vi "CRYLoad Hardware Calibration.vi"() -> ()   [LabVIEW 2013]
uses:
  CRYSystem/Typedef Control/CRYStep.ctl
  CRYSystem/Typedef Control/CRYCalibration 2DCluster.ctl
  CRYSystem/Typedef Control/CRYCalibration Cluster.ctl
  CRYSystem/Typedef Control/CRYData Cluster.ctl
  CRYProject Editor Global.vi
  CRYMainGlobal.vi
panel:
  in  "Step":T1 {"Repeat State Array"."Start" format="%#_5g"; "Y dB ref" format="%.1f"; "Y data" items=["dB", "Lin"]; "Start" format="%#_5g"}
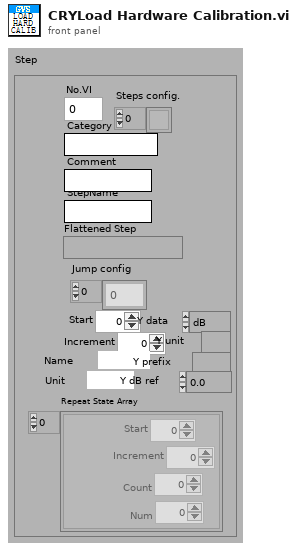
[diagram p1: front panel]
types:
  T1 = typedef "CRYStep.ctl" = cluster{"No.VI":i32, "Category":string, "StepName":string, "Seq setup flattened":string, "Comment":string, "Steps config.":bool[], "Jump config":i32[], "Start":dbl, "Increment":dbl, "Name":string, "Unit":string, "Y data":u16, "Y prefix":string, "Y dB ref":dbl, "Y unit":string, "Repeat State Array":cluster{"Start":dbl, "Increment":dbl, "Count":i32, "Num":i32}[]}
  T2 = typedef "CRYCalibration All Cluster.ctl" = cluster{"Calibration 2D":T3[], "Help":string, "Tab Value":i32, "Input Signal Type":string, "Output Signal Type":string}
  T3 = typedef "CRYCalibration 2DCluster.ctl" = cluster{"Calibration":T4, "Corr Curve":T5, "EQ Curve":T5, "Sens Curve":T5}
  T4 = typedef "CRYCalibration Cluster.ctl" = cluster{"Calibration Step Name":string, "Device":string, "Correction Curve Name":string, "Equalization Curve Name":string, "Sensitivity Curve Name":string, "Corr Folder and File":string, "EQ Folder and File":string, "Sens Folder and File":string, "Corr Step size":u16, "EQ Step size":u16, "Input":bool, "Last Cal Date (sec)":timestamp, "Cha Name":string, "Corr Curve Found":bool, "EQ Curve Found":bool, "Sens Curve Found":bool, "Signal Type":string, "Calibrated Device":string, "Hz":u32}
  T5 = typedef "CRYData Cluster.ctl" = cluster{"Name":string, "Curve":cluster{"x":dbl, "y":dbl, "z":dbl}[], "X data":u16, "Y data":u16, "Z data":u16, "X axis":u16, "Y axis":u16, "Z axis":u16, "X unit":string, "Y unit":string, "Z unit":string, "X dB ref":dbl, "Y dB ref":dbl, "Z dB ref":dbl, "single val":bool, "protected":bool, "display X":bool, "display Y":bool, "display Z":bool, "Test Info":string, "Step No.":i32, "Plot Settings":cluster{"Color":u32, "Interpolation":u8, "Point Style":u8, "Line Style":u8, "Point Color":u32, "Line Width":u8, "Bar Plot Style":u8, "Fill To":i16}, "AutoProtect":bool}
  T6 = cluster{"Signal Type":string, "Calibrated Device":string, "Cha Name":string, "Input":bool}[]
  T7 = typedef "CRYHardware.ctl" = cluster{"Name":string, "Analog I/O":u16, "Digital I/O":u16, "Channels":u8, "Dig Dev ID":u8, "N ports":u8, "Interface":u32, "Dig I/O Ports":cluster{"port #":i16, "width":i16, "direction":i32}[], "Interf settings":cluster{"Type":u16, "COM Port":u8, "Baud rate":u32, "Data bits":u32, "Parity":u16, "Stop bits":u16, "Flow control":u16, "Dev ID IEEE":u8}[], "N interfs":i32, "udev SNs":i16[], "udev enable":bool, "Channel Array":T8[], "Cal sequence":string, "SelectedIn":u16, "SelectedOut":u16, "SelectedTab":u16, "State":bool, "Help":string, "Advanced":bool, "In Audio Driver":u16, "Out Audio Driver":u16}
  T8 = typedef "CRYHardware Channel Info.ctl" = cluster{"ID":i32, "Name":string, "Digital":bool, "Input":bool, "Device Name":string, "Hardware Ch ID":u8, "Vmax (V)":dbl, "Latency (samples)":dbl, "Sampling Rate (Hz)":u32, "Bit Depth":u32, "Anti-aliasing Factor (%fs)":sgl, "DAQmx Channel":tag, "term config":i32, "Coupling":i32, "IEPE en":bool, "ASIOChannel Name":string, "Audio Driver":u16, "ASIOChannel Index":u8}
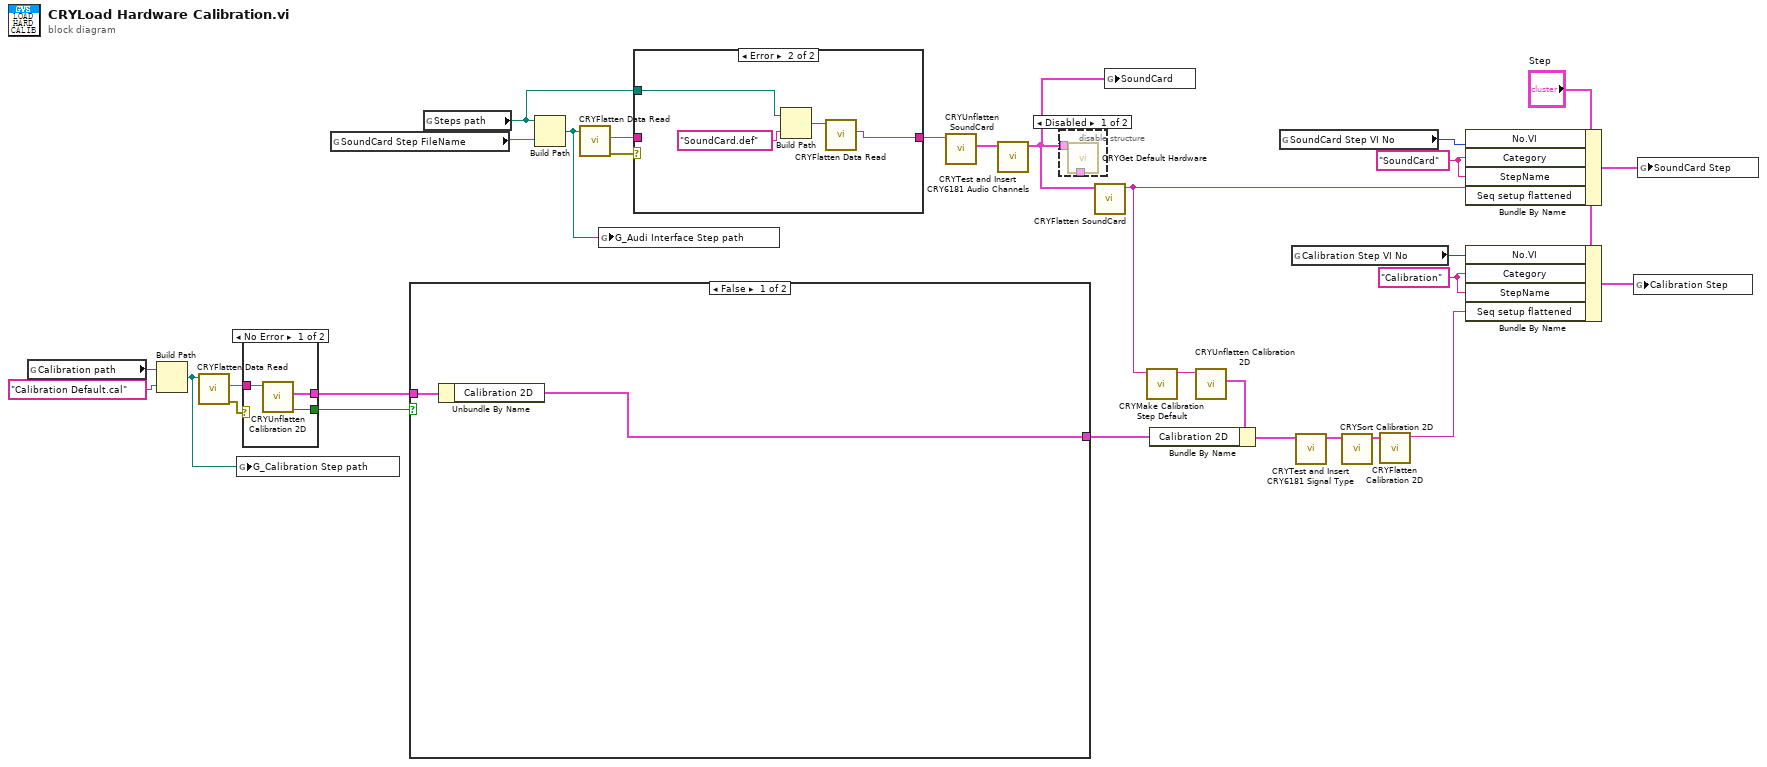
[diagram p0: block diagram]
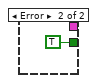
[diagram p4: hidden frame]
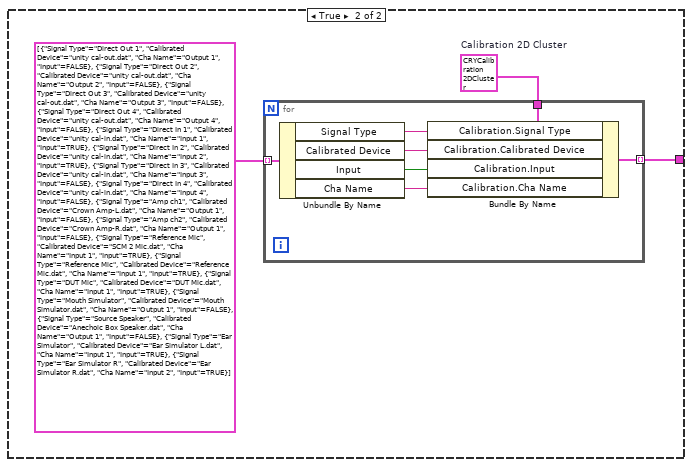
[diagram p5: hidden frame]
diagram:
  w30 = "Calibration" ("CategoryName")
  w29 = "SoundCard" ("CategoryName")
  n1 = global read "CRYMainGlobal.vi" "Calibration path"() -> (w14:path)
  n2 = Build Path(base path=w14, name or relative path="Calibration Default.cal") -> (appended path=w8:path)
  n3 = call "CRYFlatten Data Read.vi"("Path In"=w8) -> ("error out"=w15:errorcluster, "Flatten Data Out"=w19:string)  [unwired: 6 in, 1 out]
  n4 = global write "CRYProject Editor Global.vi" "G_Calibration Step path"(w8) -> ()
  n5 = case shown="No Error" w15 {
    tunnel: w19 -> [w33 _]
    tunnel: [w32 TRUE ("Error?")] -> w18
    tunnel: [w31 _] -> w17
    frame No Error {
      n6 = call "CRYUnflatten Calibration 2D.vi"("Flattened Calibration"=w33) -> ("Error?"=w32:bool, "Calibration Step Out"=w31:T2)  [unwired: 2 in, 7 out]
    }
    frame Error {
    }
  }
  n7 = global read "CRYMainGlobal.vi" "SoundCard Step FileName"() -> (w1:string)
  n8 = case shown="False" w18 {
    tunnel: w17 -> [w36 _]
    tunnel: [w35 w37] -> w16
    frame False {
      n9 = Unbundle By Name(w36) -> ("Calibration 2D"=w35:T3[])
    }
    frame True {
      w39 = T3 {"Calibration"={"Calibration Step Name"="", "Device"="", "Correction Curve Name"="", "Equalization Curve Name"="", "Sensitivity Curve Name"="", "Corr Folder and File"="", "EQ Folder and File"="", "Sens Folder and File"="", "Corr Step size"=0, "EQ Step size"=0, "Input"=FALSE, "Last Cal Date (sec)"=timestamp(0 s since 1904-01-01), "Cha Name"="", "Corr Curve Found"=FALSE, "EQ Curve Found"=FALSE, "Sens Curve Found"=FALSE, "Signal Type"="", "Calibrated Device"="", "Hz"=0}, "Corr Curve"={"Name"="", "Curve"=[], "X data"=1, "Y data"=1, "Z data"=1, "X axis"=0, "Y axis"=1, "Z axis"=1, "X unit"="Hz", "Y unit"="", "Z unit"="deg.", "X dB ref"=1.0, "Y dB ref"=1.0, "Z dB ref"=1.0, "single val"=FALSE, "protected"=FALSE, "display X"=TRUE, "display Y"=TRUE, "display Z"=TRUE, "Test Info"="", "Step No."=0, "Plot Settings"={"Color"=0, "Interpolation"=0, "Point Style"=0, "Line Style"=0, "Point Color"=0, "Line Width"=0, "Bar Plot Style"=0, "Fill To"=0}, "AutoProtect"=FALSE}, "EQ Curve"={"Name"="", "Curve"=[], "X data"=1, "Y data"=1, "Z data"=1, "X axis"=0, "Y axis"=1, "Z axis"=1, "X unit"="Hz", "Y unit"="", "Z unit"="deg.", "X dB ref"=1.0, "Y dB ref"=1.0, "Z dB ref"=1.0, "single val"=FALSE, "protected"=FALSE, "display X"=TRUE, "display Y"=TRUE, "display Z"=TRUE, "Test Info"="", "Step No."=0, "Plot Settings"={"Color"=0, "Interpolation"=0, "Point Style"=0, "Line Style"=0, "Point Color"=0, "Line Width"=0, "Bar Plot Style"=0, "Fill To"=0}, "AutoProtect"=FALSE}, "Sens Curve"={"Name"="", "Curve"=[], "X data"=1, "Y data"=1, "Z data"=1, "X axis"=0, "Y axis"=1, "Z axis"=1, "X unit"="Hz", "Y unit"="", "Z unit"="deg.", "X dB ref"=1.0, "Y dB ref"=1.0, "Z dB ref"=1.0, "single val"=FALSE, "protected"=FALSE, "display X"=TRUE, "display Y"=TRUE, "display Z"=TRUE, "Test Info"="", "Step No."=0, "Plot Settings"={"Color"=0, "Interpolation"=0, "Point Style"=0, "Line Style"=0, "Point Color"=0, "Line Width"=0, "Bar Plot Style"=0, "Fill To"=0}, "AutoProtect"=FALSE}}  # Calibration 2D Cluster
      n10 = for {
        tunnel: T6 [{"Signal Type"="Direct Out 1", "Calibrated Device"="unity cal-out.dat", "Cha Name"="Output 1", "Input"=FALSE}, {"Signal Type"="Direct Out 2", "Calibrated Device"="unity cal-out.dat", "Cha Name"="Output 2", "Input"=FALSE}, {"Signal Type"="Direct Out 3", "Calibrated Device"="unity cal-out.dat", "Cha Name"="Output 3", "Input"=FALSE}, {"Signal Type"="Direct Out 4", "Calibrated Device"="unity cal-out.dat", "Cha Name"="Output 4", "Input"=FALSE}, {"Signal Type"="Direct In 1", "Calibrated Device"="unity cal-in.dat", "Cha Name"="Input 1", "Input"=TRUE}, {"Signal Type"="Direct In 2", "Calibrated Device"="unity cal-in.dat", "Cha Name"="Input 2", "Input"=TRUE}, {"Signal Type"="Direct In 3", "Calibrated Device"="unity cal-in.dat", "Cha Name"="Input 3", "Input"=FALSE}, {"Signal Type"="Direct In 4", "Calibrated Device"="unity cal-in.dat", "Cha Name"="Input 4", "Input"=FALSE}, {"Signal Type"="Amp ch1", "Calibrated Device"="Crown Amp-L.dat", "Cha Name"="Output 1", "Input"=FALSE}, {"Signal Type"="Amp ch2", "Calibrated Device"="Crown Amp-R.dat", "Cha Name"="Output 1", "Input"=FALSE}, {"Signal Type"="Reference Mic", "Calibrated Device"="SCM 2 Mic.dat", "Cha Name"="Input 1", "Input"=TRUE}, {"Signal Type"="Reference Mic", "Calibrated Device"="Reference Mic.dat", "Cha Name"="Input 1", "Input"=TRUE}, {"Signal Type"="DUT Mic", "Calibrated Device"="DUT Mic.dat", "Cha Name"="Input 1", "Input"=TRUE}, {"Signal Type"="Mouth Simulator", "Calibrated Device"="Mouth Simulator.dat", "Cha Name"="Output 1", "Input"=FALSE}, {"Signal Type"="Source Speaker", "Calibrated Device"="Anechoic Box Speaker.dat", "Cha Name"="Output 1", "Input"=FALSE}, {"Signal Type"="Ear Simulator", "Calibrated Device"="Ear Simulator L.dat", "Cha Name"="Input 1", "Input"=TRUE}, {"Signal Type"="Ear Simulator R", "Calibrated Device"="Ear Simulator R.dat", "Cha Name"="Input 2", "Input"=TRUE}] ("Array") -> [w46] mode=indexing
        tunnel: w39 -> [w45]
        tunnel: [w40] -> w37 mode=indexing
        n11 = Unbundle By Name(w46) -> ("Signal Type"=w41:string, "Calibrated Device"=w42:string, "Input"=w43:bool, "Cha Name"=w44:string)
        n12 = Bundle By Name(cluster=w45, "Calibration.Signal Type"=w41, "Calibration.Calibrated Device"=w42, "Calibration.Input"=w43, "Calibration.Cha Name"=w44) -> (w40:T3)
      }
    }
  }
  n13 = global read "CRYMainGlobal.vi" "Steps path"() -> (w11:path)
  n14 = Build Path(base path=w11, name or relative path=w1) -> (appended path=w9:path)
  n15 = call "CRYFlatten Data Read.vi"("Path In"=w9) -> ("error out"=w13:errorcluster, "Flatten Data Out"=w12:string)  [unwired: 6 in, 1 out]
  n16 = global write "CRYProject Editor Global.vi" "G_Audi Interface Step path"(w9) -> ()
  n17 = case shown="Error" w13 {
    tunnel: w12 -> [w47 _]
    tunnel: [w47 w48] -> w10
    tunnel: w11 -> [_ w50]
    frame No Error {
    }
    frame Error {
      n18 = Build Path(base path=w50, name or relative path="SoundCard.def" ("Step File Name")) -> (appended path=w49:path)
      n19 = call "CRYFlatten Data Read.vi"("Path In"=w49) -> ("Flatten Data Out"=w48:string)  [unwired: 6 in, 2 out]
    }
  }
  n20 = call "CRYUnflatten SoundCard.vi"("Flatten SoundCard"=w10) -> ("SoundCard"=w3:T7)  [unwired: 10 out]
  n21 = call "CRYTest and Insert CRY6181 Audio Channels.vi"("Hardware in"=w3) -> ("Hardware out"=w2:T7)  [unwired: 9 in, 1 out]
  n22 = disable-structure shown="Disabled" {
    disable-tunnel: [w53 _] -> _
    disable-tunnel: w2 -> [w52 _]
    frame Disabled {
      n23 = call "CRYGet Default Hardware.vi"("Hardware Cluster In"=w52) -> ("Hardware Cluster Out"=w53:T7)  [unwired: 18 out]
    }
    frame Enabled {
    }
  }
  n24 = call "CRYFlatten SoundCard.vi"("SoundCard"=w2) -> ("SoundCard flattened"=w28:string)  [unwired: 10 out]
  n25 = global write "CRYProject Editor Global.vi" "SoundCard"(w2) -> ()
  n26 = call "CRYMake Calibration Step Default.vi"("Hardware flattened"=w28) -> ("Calibration flattened"=w22:string)  [unwired: 10 in]
  n27 = call "CRYUnflatten Calibration 2D.vi"("Flattened Calibration"=w22) -> ("Calibration Step Out"=w21:T2)  [unwired: 8 in, 2 out]
  n28 = Bundle By Name(cluster=w21, "Calibration 2D"=w16) -> (w5:T2)
  n29 = global read "CRYProject Editor Global.vi" "SoundCard Step VI No"() -> (w24:i32)
  n30 = global read "CRYProject Editor Global.vi" "Calibration Step VI No"() -> (w23:i32)
  n31 = call "CRYTest and Insert CRY6181 Signal Type.vi"("Calibration In"=w5) -> ("Calibration out"=w4:T2)  [unwired: 9 in, 1 out]
  n32 = call "CRYSort Calibration 2D.vi"("Calibration In"=w4) -> ("Calibration Out"=w6:T2)  [unwired: 10 in]
  n33 = call "CRYFlatten Calibration 2D.vi"("Calibration All Cluster"=w6) -> ("Calibration flattened"=w7:string)  [unwired: 10 in]
  n34 = Bundle By Name(cluster="Step", "No.VI"=w24, "Category"=w29, "StepName"=w29, "Seq setup flattened"=w28) -> (w26:T1)
  n35 = Bundle By Name(cluster="Step", "No.VI"=w23, "Category"=w30, "StepName"=w30, "Seq setup flattened"=w7) -> (w25:T1)
  n36 = global write "CRYProject Editor Global.vi" "Calibration Step"(w25) -> ()
  n37 = global write "CRYProject Editor Global.vi" "SoundCard Step"(w26) -> ()
